vi "Send Start Message.vi"(8 "error in (no error)":errorcluster, 11 "Generic Controller in":refnum<class "Generic Plugin.lvclass">) -> (0 "error out":errorcluster, 3 "Generic Controller out":refnum<class "Generic Plugin.lvclass">)   [LabVIEW 2020, in "Generic Plugin.lvclass"]
uses:
  Generic Plugin.lvclass
  <userlib>/Dynamic Reentrant/Dynamic Reentrant.lvlib
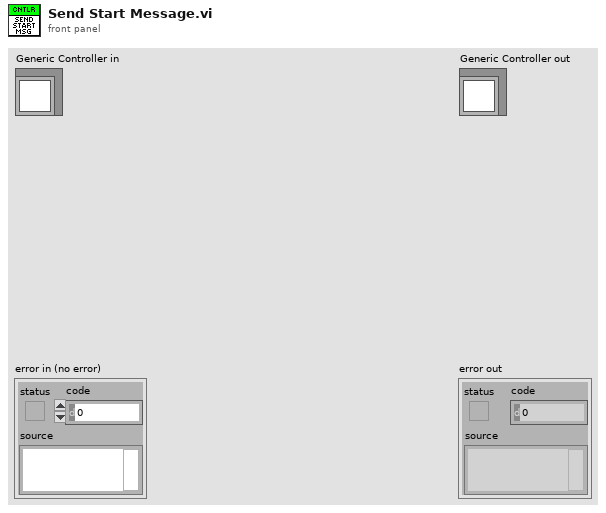
[diagram p1: front panel]
types:
  T1 = typedef "Dynamic Reentrant.lvlib/Message.ctl" = cluster{"Source":string, "Destination":string, "Time Stamp":timestamp, "Command":string, "Data":variant}
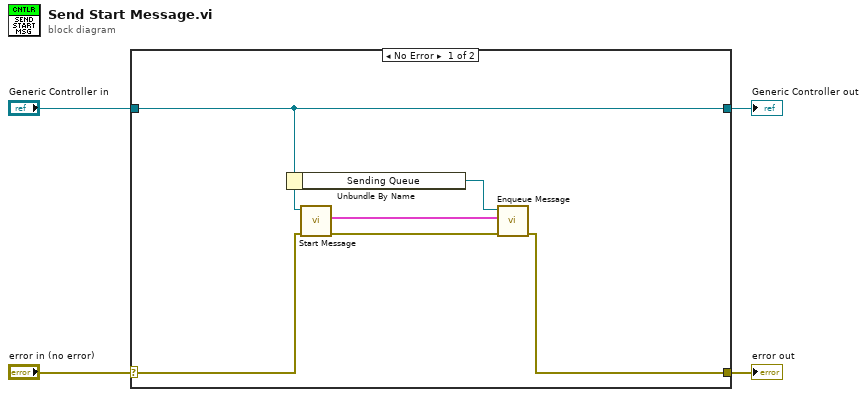
[diagram p0: block diagram]
diagram:
  n1 = case shown="No Error" "error in (no error)" {
    selector: "error in (no error)" -> [w10 w12]
    tunnel: [w5 w12] -> w3
    tunnel: [w9 w11] -> w1
    tunnel: "Generic Controller in" -> [w9 w11]
    frame No Error {
      n2 = Unbundle By Name(w9) -> ("Sending Queue"=w8:refnum<queue>)
      n3 = call-dynamic "Start Message.vi"("error in (no error)"=w10, "Generic Controller in"=w9) -> ("error out"=w6:errorcluster, "Start Message"=w7:T1)  [unwired: 7 in, 1 out]
      n4 = call <userlib>:"Enqueue Message.vi"("error in (no error)"=w6, "Message"=w7, "Listening Queue"=w8) -> ("error out"=w5:errorcluster)  [unwired: 7 in, 1 out]
    }
    frame Error {
    }
  }
  "error out" <- w3
  "Generic Controller out" <- w1
